vi "AttackerNormal.vi"(7 "IA State Input 2":T2, 8 "atacando contra?":bool=TRUE, 9 "balls":T5[](array[typedef])=[{"x"=-974.5169677734375, "y"=-3444.3310546875, "timestamp"=timestamp(2082759045.994995 s since 1904-01-01), "Vel_x"=0.0, "Vel_y"=0.0, "Pos Bola Est"=[]}], 10 "Field Size in":T6={"line_width"=10, "field_length"=9000, "field_width"=6000, "boundary_width"=250, "referee_width"=425, "goal_width"=700, "goal_depth"=180, "goal_wall_width"=20, "center_circle_radius"=500, "defense_radius"=500, "defense_stretch"=350, "free_kick_from_defense_dist"=700, "penalty_spot_from_field_line_dist"=450, "penalty_line_from_spot_dist"=350}, 11 "Robot in":T3={"id"=5, "function"=enum."Attacker", "x"=-983.1382446289062, "y"=-3000.010498046875, "orientation"=-1.5516623258590698, "v_tangent"=0.0, "v_normal"=0.0, "v_ang"=0.0, "kick_x"=0.0, "kick_z"=0.0, "dribble"=FALSE, "Timestamp"=timestamp(2082759045.994995 s since 1904-01-01), "dest_x"=0.0, "dest_y"=0.0, "dest_orientation"=0.0, "estimatives"={"est_v_tangent"=0.0, "est_v_normal"=0.0, "est_vx"=0.0, "est_vy"=0.0, "Pos Robot Est"=[]}, "dest_x_kick"=0.0, "dest_y_kick"=0.0, "Gap Coord"=[], "States"=enum."GoToTangent"}) -> (1 "Next State":T1=enum."GoToTangent", 2 "Robot out":T3={"id"=5, "function"=enum."Attacker", "x"=-983.1382446289062, "y"=-3000.010498046875, "orientation"=-1.5516623258590698, "v_tangent"=0.0001540345015520423, "v_normal"=0.008599927144915481, "v_ang"=0.002668461263266586, "kick_x"=0.0, "kick_z"=0.0, "dribble"=FALSE, "Timestamp"=timestamp(2082759045.994995 s since 1904-01-01), "dest_x"=0.0, "dest_y"=0.0, "dest_orientation"=0.0, "estimatives"={"est_v_tangent"=0.0, "est_v_normal"=0.0, "est_vx"=0.0, "est_vy"=0.0, "Pos Robot Est"=[]}, "dest_x_kick"=0.0, "dest_y_kick"=0.0, "Gap Coord"=[], "States"=enum."GoToTangent"}, 6 "Current States":T1=enum."GoToTangent")   [LabVIEW 2016]
uses:
  Core/AI Robot.ctl
  Functions Enum.ctl
  AttackerStates.ctl
  Core/Field Size.ctl
  Core/AI Ball.ctl
  Core/AI Input.ctl
  Core/AI Judge.ctl
  Command Enum.ctl
  Util/Events/Events.ctl
panel:
  out "Boolean":bool
  in  "Kick Force":dbl=100.0 format="%#_13g"
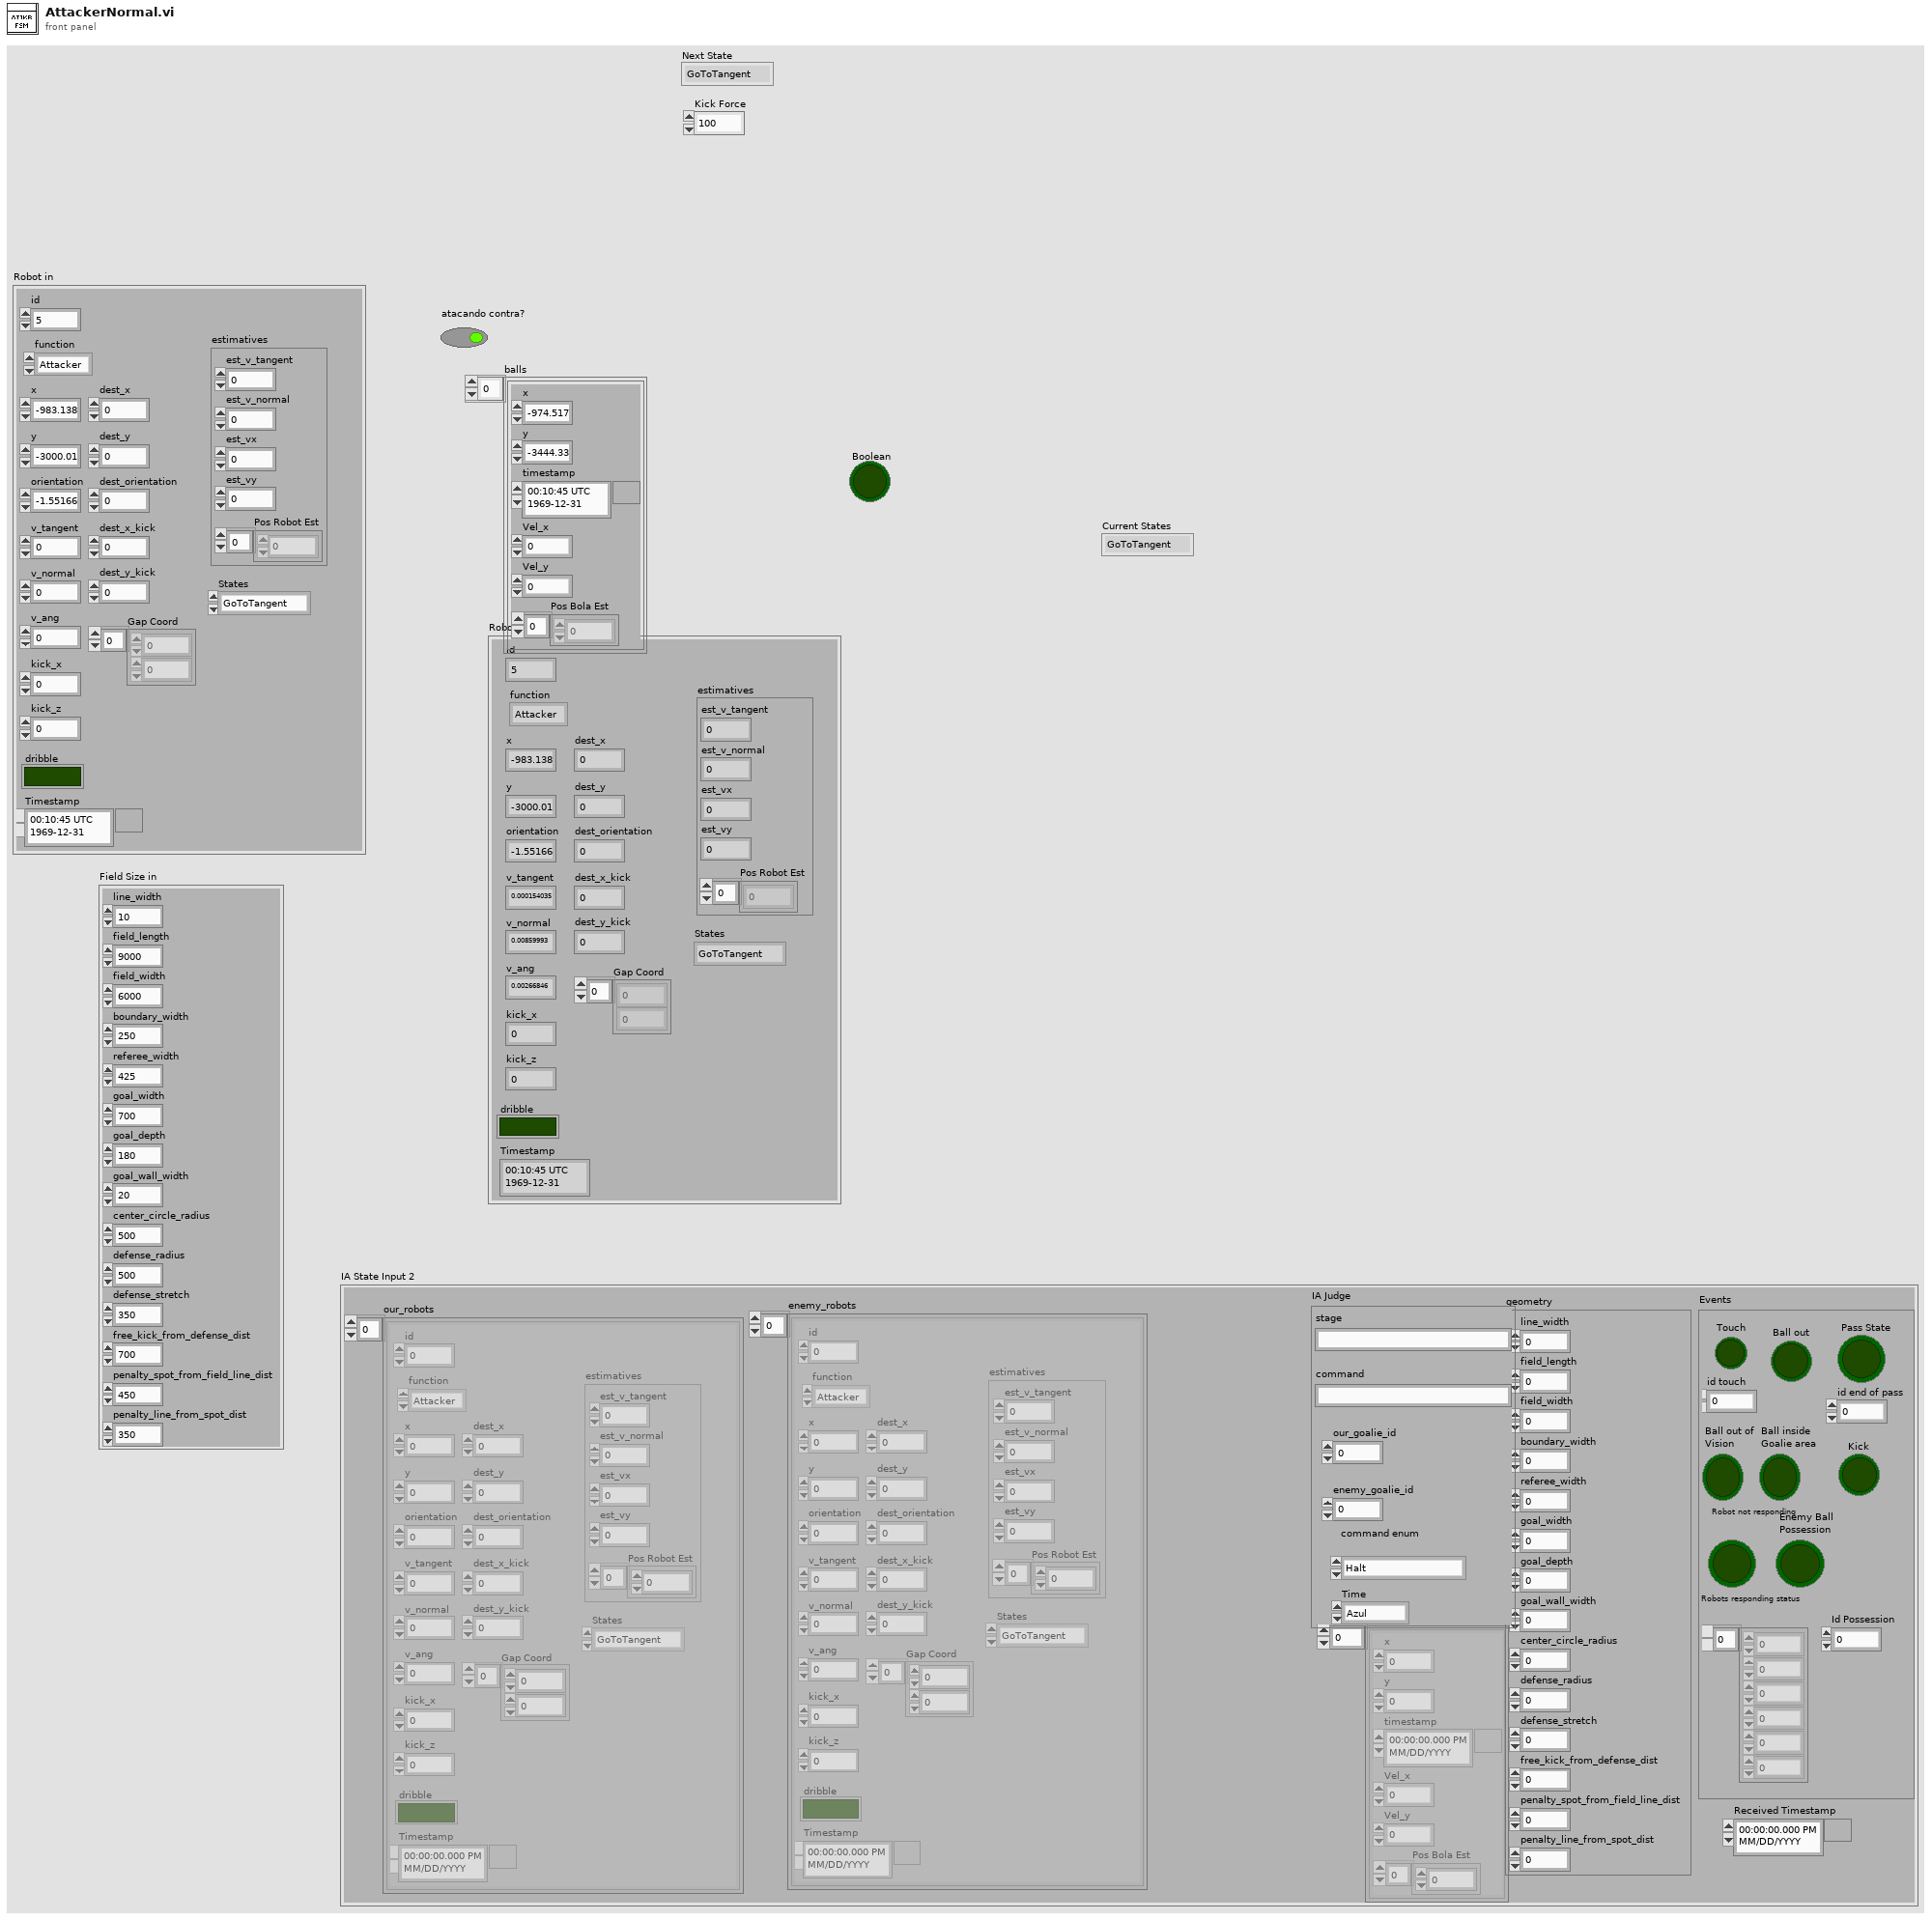
[diagram p1: front panel]
types:
  T1 = typedef "AttackerStates.ctl" = enum16{"Pass", "GoToTangent", "BallGetting", "GoToKick", ""}
  T2 = typedef "AI Input.ctl" = cluster{"our_robots":T3[], "enemy_robots":T3[], "balls":T5[], "geometry":T6, "IA Judge":T7, "Received Timestamp":timestamp, "Events":T9}
  T3 = typedef "AI Robot.ctl" = cluster{"id":u32, "function":T4, "x":dbl, "y":dbl, "orientation":dbl, "v_tangent":dbl, "v_normal":dbl, "v_ang":dbl, "kick_x":dbl, "kick_z":dbl, "dribble":bool, "Timestamp":timestamp, "dest_x":dbl, "dest_y":dbl, "dest_orientation":dbl, "estimatives":cluster{"est_v_tangent":dbl, "est_v_normal":dbl, "est_vx":dbl, "est_vy":dbl, "Pos Robot Est":dbl[]}, "dest_x_kick":dbl, "dest_y_kick":dbl, "Gap Coord":dbl[], "States":T1}
  T4 = typedef "Functions Enum.ctl" = enum16{"Attacker", "Goalie", "Defender", "Striker", "Goto 0", "Dummy", "Kicker", "ZigZag"}
  T5 = typedef "AI Ball.ctl" = cluster{"x":dbl, "y":dbl, "timestamp":timestamp, "Vel_x":dbl, "Vel_y":dbl, "Pos Bola Est":dbl[]}
  T6 = typedef "Field Size.ctl" = cluster{"line_width":u32, "field_length":u32, "field_width":u32, "boundary_width":u32, "referee_width":u32, "goal_width":u32, "goal_depth":u32, "goal_wall_width":u32, "center_circle_radius":u32, "defense_radius":u32, "defense_stretch":u32, "free_kick_from_defense_dist":u32, "penalty_spot_from_field_line_dist":u32, "penalty_line_from_spot_dist":u32}
  T7 = typedef "AI Judge.ctl" = cluster{"stage":string, "command":string, "our_goalie_id":dbl, "enemy_goalie_id":dbl, "command enum":T8, "Time":enum16{"Azul", "Amarelo"}}
  T8 = typedef "Command Enum.ctl" = enum16{"Halt", "Stop", "Force Start", "PKA Normal Start", "Prepare Kickoff Ally", "PKE Normal Start", "Prepare Kickoff Enemy", "Prepare Penalty Ally", "PPA Normal Start", "Prepare Penalty Enemy", "PPE Normal Start", "Direct Free Enemy", "Direct Free Ally", "Indirect Free Enemy", "Indirect Free Ally", "Timeout Enemy", "Timeout Ally", "Goal Enemy", "Goal Ally", "Ball Placement Enemy", "Ball Placement Ally", "Normal Half Time", "Extra Time Break", "Extra Half Time", "None"}
  T9 = typedef "Events.ctl" = cluster{"Touch":bool, "Ball out":bool, "id touch":dbl, "Ball out of \nVision":bool, "Ball inside \nGoalie area":bool, "Robot not responding":bool, "Robots responding status":dbl[], "Enemy Ball \nPossession":bool, "Pass State":bool, "id end of pass":dbl, "Kick":bool, "Id Possession":dbl}
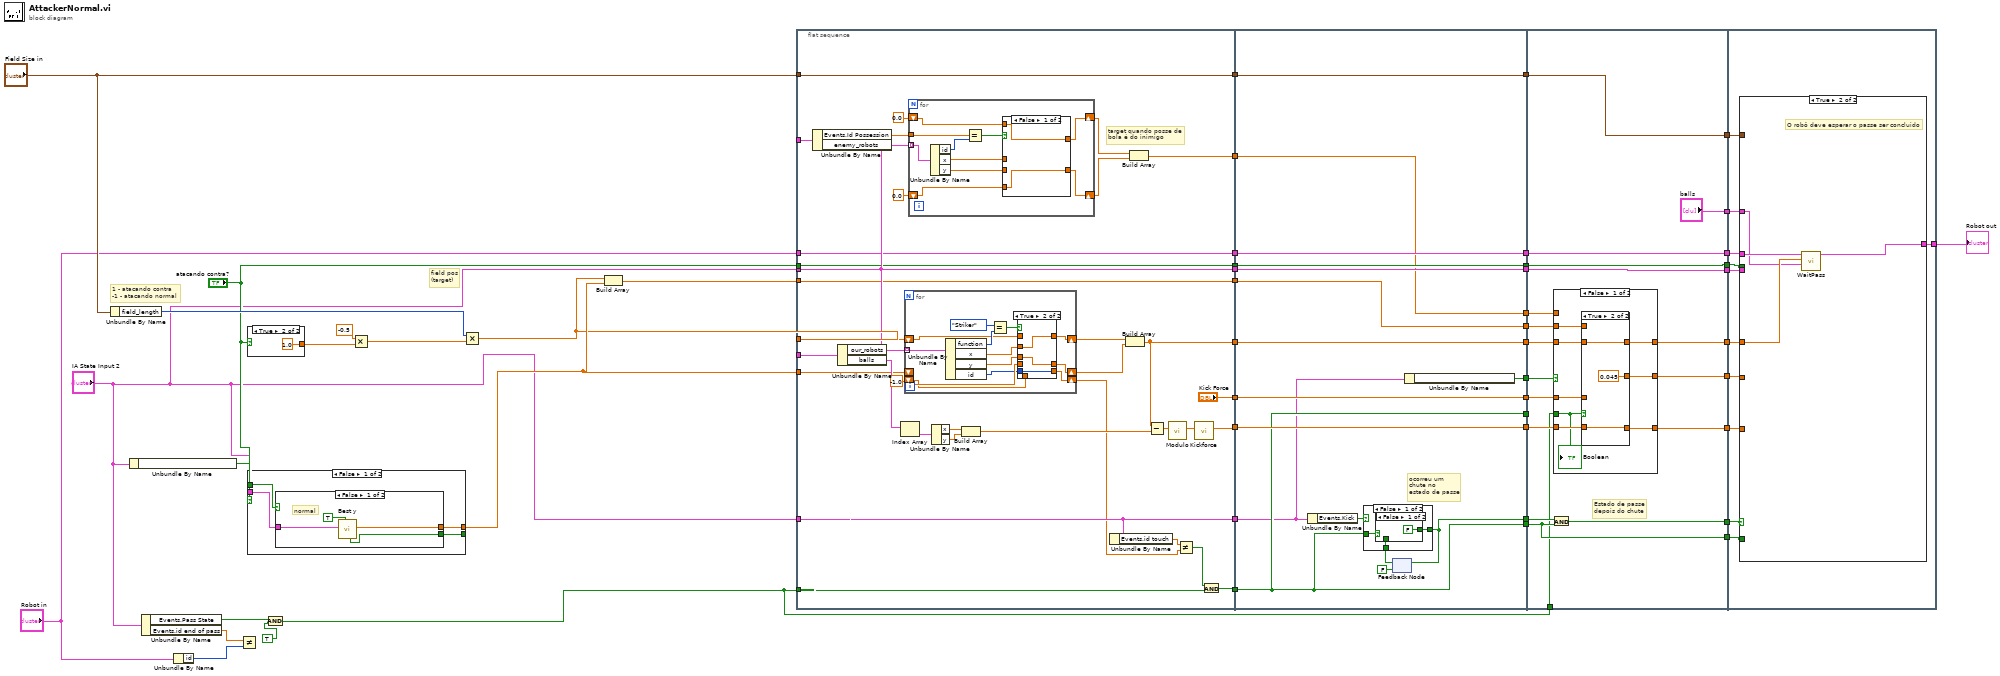
[diagram p0: block diagram]
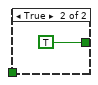
[diagram p5: hidden frame]
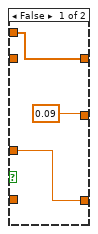
[diagram p6: hidden frame]
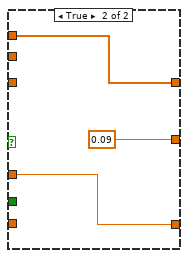
[diagram p7: hidden frame]
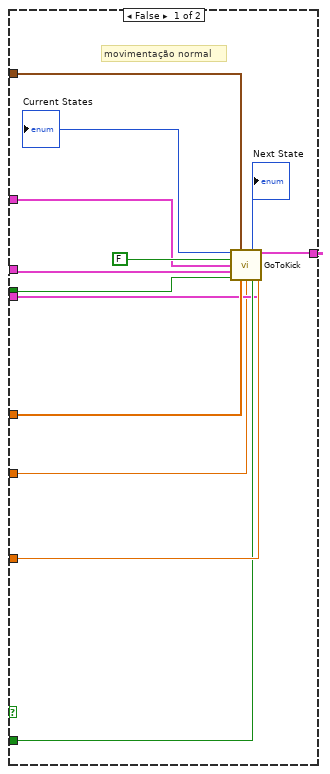
[diagram p8: hidden frame]
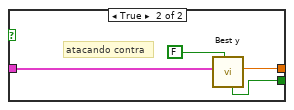
[diagram p9: hidden frame]
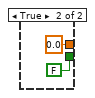
[diagram p10: hidden frame]
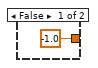
[diagram p11: hidden frame]
diagram:
  # "1 - atacando contra\n-1 - atacando normal"
  # "field pos\n(target)"
  n1 = Unbundle By Name("Field Size in") -> ("field_length"=w52:u32)
  n2 = Unbundle By Name("IA State Input 2") -> ("Events.Ball inside \nGoalie area"=w48:bool)
  n3 = Unbundle By Name("IA State Input 2") -> ("Events.Pass State"=w42:bool, "Events.id end of pass"=w44:dbl)
  n4 = Unbundle By Name("Robot in") -> ("id"=w43:u32)
  n5 = Not Equal?(x=w44, y=w43) -> ()  [unwired: 1 out]
  n6 = case shown="True" "atacando contra?" {
    tunnel: [-1.0 ("attck contra? 2") 1.0] -> w49
    frame False {
    }
    frame True {
    }
  }
  n7 = case shown="False" w48 {
    tunnel: "atacando contra?" -> [w58 _]
    tunnel: [w57 0.0] -> w20
    tunnel: "IA State Input 2" -> [w56 _]
    tunnel: [w55 FALSE ("Eclipse")] -> _
    frame False {
      n8 = case shown="False" w58 {
        tunnel: [w61 w65] -> w57
        tunnel: w56 -> [w59 w64]
        tunnel: [w60 w63] -> w55
        frame False {
          # "normal"
          n9 = call "Best y.vi"("inimigos"=TRUE, "IA State"=w59) -> ("Best y"=w61:dbl, "Eclipse"=w60:bool)  [unwired: 6 in, 2 out]
        }
        frame True {
          # "atacando contra"
          n10 = call "Best y.vi"("inimigos"=FALSE, "IA State"=w64) -> ("Best y"=w65:dbl, "Eclipse"=w63:bool)  [unwired: 6 in, 2 out]
        }
      }
    }
    frame True {
    }
  }
  n11 = And(x=w42, y=TRUE) -> (x .and. y?=w2:bool)
  n12 = Multiply(x=-0.5, y=w49) -> (x*y=w50:dbl)
  n13 = Multiply(x=w52, y=w50) -> (x*y=w19:dbl)
  n14 = Build Array(w19, w20) -> (w41:dbl[])
  n15 = flat-sequence {
    tunnel: "IA State Input 2" -> [w82]
    tunnel: w2 -> [w78]
    tunnel: w19 -> [w84]
    tunnel: w41 -> [w100]
    tunnel: "IA State Input 2" -> [w101]
    tunnel: "Robot in" -> [w102]
    tunnel: "Field Size in" -> [w103]
    tunnel: "atacando contra?" -> [w104]
    tunnel: [w104] -> w29
    tunnel: [w103] -> w28
    tunnel: [w102] -> w27
    tunnel: [w101] -> w26
    tunnel: [w86] -> w25
    tunnel: [w100] -> w24
    tunnel: [w87] -> w23
    tunnel: [w77] -> w22
    tunnel: [w82] -> w21
    tunnel: w20 -> [w89]
    tunnel: "IA State Input 2" -> [w88]
    tunnel: ["Kick Force"] -> w18
    tunnel: "IA State Input 2" -> [w76]
    tunnel: [w71] -> w13
    tunnel: [w153] -> w40
    tunnel: [w152] -> w39
    tunnel: [w151] -> w38
    tunnel: [w150] -> w37
    tunnel: [w142] -> w36
    tunnel: [w149] -> w35
    tunnel: [w148] -> w34
    tunnel: [w147] -> w33
    tunnel: [w146] -> w32
    tunnel: [w141] -> w31
    tunnel: [w141] -> w30
    tunnel: w29 -> [w153]
    tunnel: w28 -> [w152]
    tunnel: w27 -> [w151]
    tunnel: w26 -> [w150]
    tunnel: w25 -> [w148]
    tunnel: w24 -> [w147]
    tunnel: w23 -> [w146]
    tunnel: w22 -> [w141]
    tunnel: w21 -> [w140]
    tunnel: w18 -> [w149]
    tunnel: [w139] -> w16
    tunnel: [w138] -> w14
    tunnel: w13 -> [w138]
    tunnel: w40 -> [w167]
    tunnel: w39 -> [w170]
    tunnel: w38 -> [w169]
    tunnel: w37 -> [w168]
    tunnel: w36 -> [w177]
    tunnel: w35 -> [w176]
    tunnel: w34 -> [w175]
    tunnel: w33 -> [w174]
    tunnel: w32 -> [w173]
    tunnel: w31 -> [w162]
    tunnel: w30 -> [_]
    tunnel: w16 -> [w172]
    tunnel: w14 -> [w171]
    tunnel: [w170] -> w12
    tunnel: [w169] -> w11
    tunnel: [w168] -> w10
    tunnel: [w167] -> w9
    tunnel: [w166] -> w8
    tunnel: [w165] -> w7
    tunnel: [w164] -> w6
    tunnel: [w163] -> w5
    tunnel: [w162] -> w4
    tunnel: w2 -> [w161]
    tunnel: ["balls"] -> w1
    tunnel: w12 -> [w205]
    tunnel: w11 -> [w204]
    tunnel: w10 -> [w203]
    tunnel: w9 -> [w202]
    tunnel: w8 -> [w201]
    tunnel: w7 -> [w200]
    tunnel: w6 -> [w199]
    tunnel: w5 -> [w198]
    tunnel: w4 -> [w197]
    tunnel: [w196] -> w3
    tunnel: w1 -> [w195]
    frame #0 {
      # "target quando posse de\nbola é do inimigo"
      n16 = Unbundle By Name(w76) -> ("Events.Id Possession"=w74:dbl, "enemy_robots"=w75:T3[])
      n17 = Unbundle By Name(w88) -> ("our_robots"=w90:T3[], "balls"=w93:T5[])
      n18 = Index Array(array=w93) -> (element=w94:T5)  [unwired: 1 in]
      n19 = for {
        tunnel: w90 -> [w131] mode=indexing
        shift-right: [w126] -> w91
        shift-left: w84 -> [w125]
        shift-right: [w123] -> w92
        shift-left: w89 -> [w122]
        shift-right: [w120] -> w80
        shift-left: -1.0 -> [w119]
        n20 = Unbundle By Name(w131) -> ("function"=w130:T4, "x"=w127:dbl, "y"=w124:dbl, "id"=w121:u32)
        n21 = Equal?(x=Functions_Enum."Striker", y=w130) -> (x = y?=w128:bool)
        n22 = case shown="True" w128 {
          tunnel: [w134 w137] -> w126
          tunnel: w127 -> [_ w137]
          tunnel: w125 -> [w134 _]
          tunnel: w124 -> [_ w136]
          tunnel: [w133 w136] -> w123
          tunnel: w122 -> [w133 _]
          tunnel: w121 -> [_ w135]
          tunnel: [w132 w135] -> w120
          tunnel: w119 -> [w132 _]
          frame False {
          }
          frame True {
          }
        }
      }
      n23 = for {
        tunnel: w75 -> [w114] mode=indexing
        tunnel: w74 -> [w112]
        shift-right: [w108] -> w73
        shift-left: 0.0 ("x") -> [w106]
        shift-right: [w107] -> w72
        shift-left: 0.0 ("y") -> [w105]
        n24 = Unbundle By Name(w114) -> ("id"=w113:u32, "x"=w110:dbl, "y"=w109:dbl)
        n25 = Equal?(x=w112, y=w113) -> (x = y?=w111:bool)
        n26 = case shown="False" w111 {
          tunnel: w110 -> [_ w118]
          tunnel: w109 -> [_ w117]
          tunnel: [w116 w118] -> w108
          tunnel: [w115 w117] -> w107
          tunnel: w106 -> [w116 _]
          tunnel: w105 -> [w115 _]
          frame False {
          }
          frame True {
          }
        }
      }
      n27 = Unbundle By Name(w94) -> ("x"=w95:dbl, "y"=w96:dbl)
      n28 = Build Array(w95, w96) -> (w97:dbl[])
      n29 = Unbundle By Name(w82) -> ("Events.id touch"=w81:dbl)
      n30 = Build Array(w91, w92) -> (w87:dbl[])
      n31 = Build Array(w73, w72) -> (w71:dbl[])
      n32 = Subtract(x=w87, y=w97) -> (x-y=w98:dbl[])
      n33 = call "Modulo.vi"("2D vector"=w98) -> ("Modulo"=w99:dbl)  [unwired: 10 in]
      n34 = Not Equal?(x=w81, y=w80) -> (x != y?=w79:bool)
      n35 = call "Kickforce.vi"("Distância ao\nalvo do chute"=w99) -> ("Força do chute"=w86:dbl)  [unwired: 9 in, 1 out]
      n36 = And(x=w79, y=w78) -> (x .and. y?=w77:bool)
    }
    frame #1 {
      # "ocorreu um \nchute no\nestado de passe"
      n37 = Unbundle By Name(w140) -> ("Events.Kick"=w143:bool)
      n38 = feedback #1(FALSE) -> (w144:bool)
      n39 = case shown="False" w143 {
        tunnel: [w155 TRUE] -> w142
        tunnel: w144 -> [w154 _]
        tunnel: w141 -> [w156 _]
        frame False {
          n40 = case shown="False" w156 {
            tunnel: [FALSE w158] -> w155
            tunnel: w154 -> [_ w158]
            frame False {
            }
            frame True {
            }
          }
        }
        frame True {
        }
      }
      n41 = feedback-in #1(w142) -> ()
      n42 = Unbundle By Name(w140) -> ("Events.Enemy Ball \nPossession"=w139:bool)
    }
    frame #2 {
      # "Estado de passe\ndepois do chute"
      n43 = And(x=w177, y=w162) -> (x .and. y?=w163:bool)
      n44 = case shown="False" w172 {
        tunnel: w176 -> [w185 w194]
        tunnel: w175 -> [w184 _]
        tunnel: w174 -> [w183 _]
        tunnel: w173 -> [w182 _]
        tunnel: [w181 w193] -> w166
        tunnel: [w180 w194] -> w164
        tunnel: w161 -> [w179 _]
        tunnel: w171 -> [_ w193]
        tunnel: [w178 0.09] -> w165
        frame False {
          n45 = case shown="True" w179 {
            tunnel: w185 -> [w187 _]
            tunnel: w184 -> [_ w190]
            tunnel: w183 -> [w188 _]
            tunnel: w182 -> [_ w191]
            tunnel: [w188 w191] -> w181
            tunnel: [w187 w190] -> w180
            tunnel: [0.09 0.045] -> w178
            frame False {
            }
            frame True {
            }
          }
          "Boolean" <- w179
        }
        frame True {
        }
      }
    }
    frame #3 {
      n46 = case shown="True" w198 {
        tunnel: w202 -> [w216 _]
        tunnel: w205 -> [w215 _]
        tunnel: w204 -> [w214 w221]
        tunnel: w201 -> [w213 w220]
        tunnel: w199 -> [w212 _]
        tunnel: w197 -> [w211 _]
        tunnel: w203 -> [w210 _]
        tunnel: [w209 w222] -> w196
        tunnel: w200 -> [w207 _]
        tunnel: w195 -> [w206 w219]
        frame False {
          # "movimentação normal"
          n47 = call "GoToKick.vi"("Field Size in"=w215, "goleiro?"=FALSE, "balls"=w206, "Robot in in"=w214, "Kick Force"=w212, "atacando contra?"=w216, "Target"=w213, "Cone de chute"=w207, "Passe"=w211, "IA State Input in"=w210) -> ("Current States"=→"Current States":T1, "Next State"=→"Next State":T1, "Robot out"=w209:T3)  [unwired: 3 in]
        }
        frame True {
          # "O robô deve esperar o passe ser concluido"
          n48 = call "WaitPass.vi"("balls"=w219, "Target"=w220, "Robot in"=w221) -> ("Robot out"=w222:T3)  [unwired: 8 in]
        }
      }
    }
  }
  "Robot out" <- w3
